vi "Reverse Tank.vi"(9 "Toggle Button":bool, 10 "Right Motor":dbl, 11 "Left Motor":dbl) -> (2 "Right Motor":dbl, 3 "Left Motor":dbl)   [LabVIEW 2011]
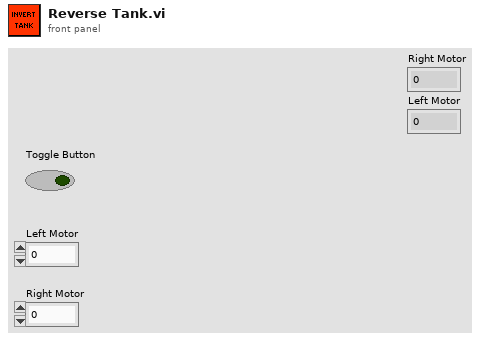
[diagram p1: front panel]
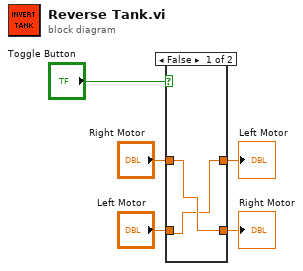
[diagram p0: block diagram]
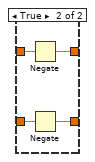
[diagram p2: hidden frame]
diagram:
  n1 = case shown="False" "Toggle Button" {
    tunnel: "Left Motor" -> [w6 w11]
    tunnel: [w7 w10] -> w4
    tunnel: [w6 w9] -> w3
    tunnel: "Right Motor" -> [w7 w8]
    frame False {
    }
    frame True {
      n2 = Negate(x=w8) -> (-x=w9:dbl)
      n3 = Negate(x=w11) -> (-x=w10:dbl)
    }
  }
  "Right Motor" <- w4
  "Left Motor" <- w3
